vi "DriveModeStateController.vi"(1 "Selected State (In)":string) -> (0 "Drive Mode":T1(ring))   [LabVIEW 2019]
uses:
  dsinstructions.vi
  sensors.vi
  dsdata.vi
  outputs.vi
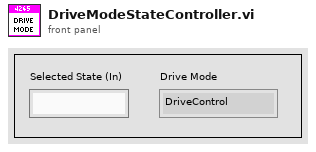
[diagram p1: front panel]
types:
  T1 = enum16{"DriveControl", "TargetControlH", "FeederStation"}
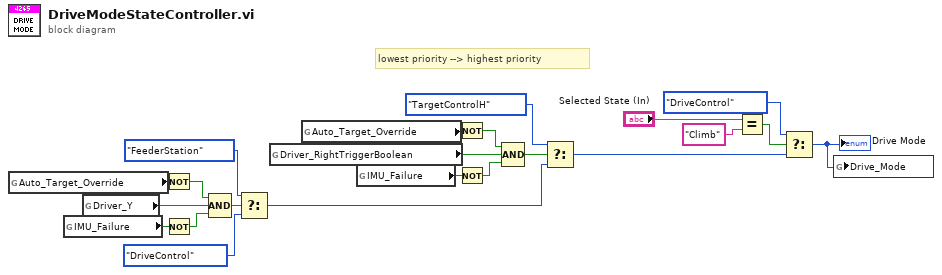
[diagram p0: block diagram]
diagram:
  # "lowest priority --> highest priority"
  n1 = global read "dsdata.vi" "Auto_Target_Override"() -> (w6:bool)
  n2 = global read "sensors.vi" "IMU_Failure"() -> (w4:bool)
  n3 = global read "dsinstructions.vi" "Driver_Y"() -> (w7:bool)
  n4 = Not(x=w6) -> (.not. x?=w5:bool)
  n5 = Not(x=w4) -> (.not. x?=w3:bool)
  n6 = Compound Arithmetic op=AND(w5, w7, w3) -> (w2:bool)
  n7 = Select(t=T1."FeederStation", s=w2, f=T1."DriveControl") -> (s? t:f=w20:T1)
  n8 = global read "dsinstructions.vi" "Driver_RightTriggerBoolean"() -> (w17:bool)
  n9 = global read "dsdata.vi" "Auto_Target_Override"() -> (w13:bool)
  n10 = global read "sensors.vi" "IMU_Failure"() -> (w11:bool)
  n11 = Not(x=w13) -> (.not. x?=w12:bool)
  n12 = Not(x=w11) -> (.not. x?=w10:bool)
  n13 = Compound Arithmetic op=AND(w12, w17, w10) -> (w1:bool)
  n14 = Select(t=T1."TargetControlH", s=w1, f=w20) -> (s? t:f=w21:T1)
  n15 = Equal?(x="Selected State (In)", y="Climb") -> (x = y?=w16:bool)
  n16 = Select(t=T1."DriveControl", s=w16, f=w21) -> (s? t:f=w22:T1)
  "Drive Mode" <- w22
  n17 = global write "outputs.vi" "Drive_Mode"(w22) -> ()
